vi "Data_split.vi"() -> ()   [LabVIEW 2021]
uses:
  <vilib>/Utility/file.llb/Read Delimited Spreadsheet (DBL).vi
  <vilib>/Utility/file.llb/Write Delimited Spreadsheet (DBL).vi
  <vilib>/gmath/NI_Gmath.lvlib
panel:
  in  "book number":i32=333
  in  "file path (dialog if empty)":path=path "\\\\ad.uillinois.edu\\engr/mrl-dvh-research/Guang Yue/data/Contour plot"
  in  "Ignore points":i32=250
  in  "Voltage treshold":dbl=-4.4e-06 format="%_3g"
  out "Ready?":bool
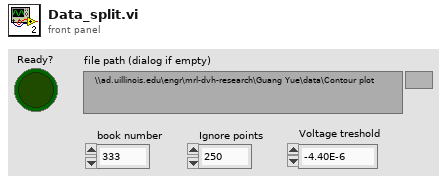
[diagram p1: front panel]
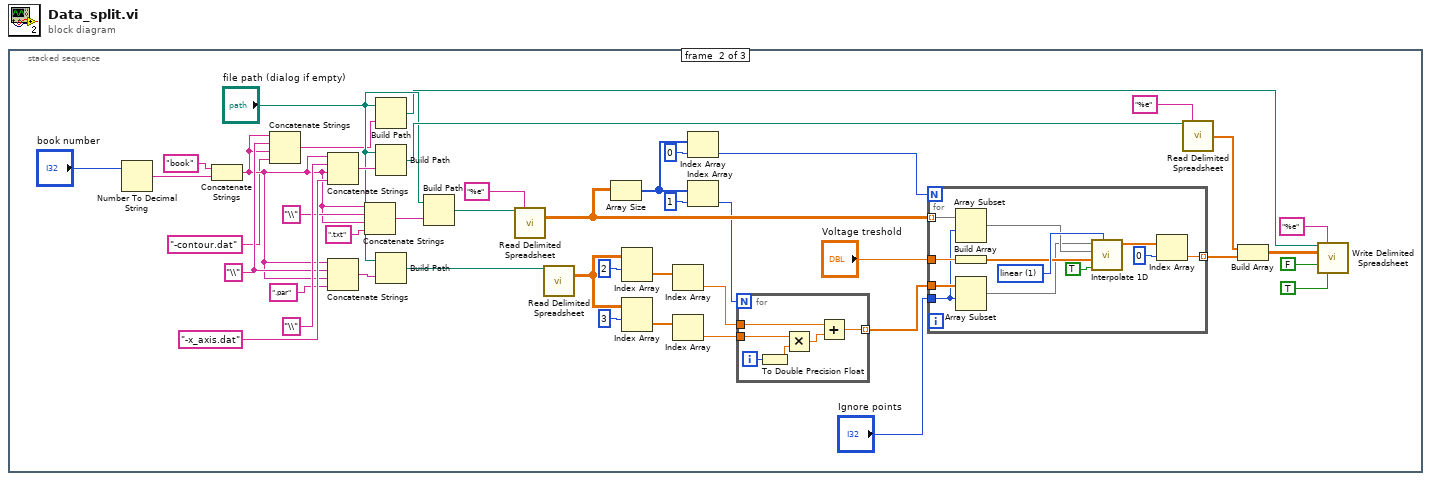
[diagram p0: block diagram]
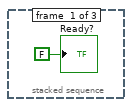
[diagram p2: hidden frame]
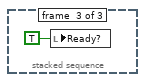
[diagram p3: hidden frame]
diagram:
  n1 = stacked-sequence {
    frame #0 {
      "Ready?" <- FALSE ("Ready?")
    }
    frame #1 {
      w13 = "\\" ("string")
      n2 = Number To Decimal String(number="book number") -> (decimal integer string=w41:string)  [unwired: 1 in]
      n3 = Concatenate Strings("book" ("string"), w41) -> (w12:string)
      n4 = Concatenate Strings(w12, w13, w12, "-contour.dat" ("string")) -> (w9:string)
      n5 = Concatenate Strings(w12, "\\" ("string"), w12, "-x_axis.dat" ("string")) -> (w23:string)
      n6 = Concatenate Strings(w12, w13, w12, ".par" ("string")) -> (w43:string)
      n7 = Concatenate Strings(w12, "\\" ("string"), w12, ".txt" ("string")) -> (w42:string)
      n8 = Build Path(base path="file path (dialog if empty)", name or relative path=w9) -> (appended path=w8:path)
      n9 = Build Path(base path="file path (dialog if empty)", name or relative path=w23) -> (appended path=w15:path)
      n10 = Build Path(base path="file path (dialog if empty)", name or relative path=w43) -> (appended path=w44:path)
      n11 = Build Path(base path="file path (dialog if empty)", name or relative path=w42) -> (appended path=w45:path)
      n12 = call-poly <vilib>:"Read Delimited Spreadsheet.vi"("file path (dialog if empty)"=w45, "format (%.3f)"="%e") -> ("all rows"=w32:dbl[][])  [unwired: 8 in, 5 out]
      n13 = call-poly <vilib>:"Read Delimited Spreadsheet.vi"("file path (dialog if empty)"=w44) -> ("all rows"=w37:dbl[][])  [unwired: 9 in, 5 out]
      n14 = Array Size(array=w32) -> (size(s)=w22:i32[])
      n15 = Index Array(array=w37, index (row)=2) -> (element=w36:dbl[])  [unwired: 1 in]
      n16 = Index Array(array=w37, index (row)=3) -> (element=w35:dbl[])  [unwired: 1 in]
      n17 = Index Array(array=w36) -> (element=w31:dbl)  [unwired: 1 in]
      n18 = Index Array(array=w35) -> (element=w30:dbl)  [unwired: 1 in]
      n19 = Index Array(array=w22, index=0) -> (element=w20:i32)
      n20 = Index Array(array=w22, index=1) -> (element=w19:i32)
      n21 = for {
        N: w19 -> [_]
        tunnel: w31 -> [w51]
        tunnel: w30 -> [w49]
        tunnel: [w47] -> w26 mode=indexing
        i -> [w50]
        n22 = To Double Precision Float(number=w50) -> (double precision float=w46:dbl)
        n23 = Multiply(x=w49, y=w46) -> (x*y=w48:dbl)
        n24 = Add(x=w51, y=w48) -> (x+y=w47:dbl)
      }
      n25 = for {
        N: w20 -> [_]
        tunnel: w32 -> [w56] mode=indexing
        tunnel: w26 -> [w57]
        tunnel: [w58] -> w3 mode=indexing
        tunnel: "Ignore points" -> [w52]
        tunnel: "Voltage treshold" -> [w53]
        w62 = 1 items=["nearest", "linear", "spline", "cubic Hermite", "Lagrange"] ("method")
        n26 = Array Subset(array=w56, index=w52) -> (w55:dbl[])  [unwired: 1 in]
        n27 = Build Array(w53) -> (w61:dbl[])
        n28 = Array Subset(array=w57, index=w52) -> (w54:dbl[])  [unwired: 1 in]
        n29 = call <vilib>:"Interpolate 1D.vi"("method"=w62, "X is monotonic"=TRUE, "xi"=w61, "X"=w55, "Y"=w54) -> ("yi"=w60:dbl[])  [unwired: 4 in, 2 out]
        n30 = Index Array(array=w60, index=0) -> (element=w58:dbl)
      }
      n31 = call-poly <vilib>:"Read Delimited Spreadsheet.vi"("file path (dialog if empty)"=w15, "format (%.3f)"="%e") -> ("first row"=w4:dbl[])  [unwired: 8 in, 5 out]
      n32 = Build Array(w4, w3) -> (w2:dbl[][])
      n33 = call-poly <vilib>:"Write Delimited Spreadsheet.vi"("file path (dialog if empty)"=w8, "format (%.3f)"="%e", "2D data"=w2, "append to file? (new file:F)"=FALSE, "transpose? (no:F)"=TRUE) -> ()  [unwired: 9 in, 2 out]
    }
    frame #2 {
      n34 = local write "Ready?"(TRUE ("Ready?")) -> ()
    }
  }
